vi "Append Control Image to Report.vi"(0 "report in":refnum<class "NI_report.lvclass">, 1 "alignment (default)":T2, 2 "image file type (.jpg)":enum16{".jpg", ".png"}(ring), 5 "image depth":T1=2 items=["B&W", "4 bits", "8 bits", "24 bits"], 7 "ctrl reference":refnum<vi>, 9 "description":string, 11 "error in (no error)":errorcluster, 12 "MS Office parameters":T3) -> (4 "report out":refnum<class "NI_report.lvclass">, 8 "start out (Word)":i32, 10 "end out (Word)":i32, 15 "error out":errorcluster)   [LabVIEW 2017, in "NI_report.lvclass"]
doc: "Creates an image of the front panel object specified in <B>ctrl reference</B> and appends it to a report."
uses:
  <vilib>/Utility/NIReport.llb/NI_report.lvclass
  <vilib>/Utility/NIReport.llb/HTML Report Image Alignment.ctl
  <vilib>/Utility/NIReport.llb/image depth.ctl
  <vilib>/Utility/NIReport.llb/NI_ReportGenerationCore.lvlib
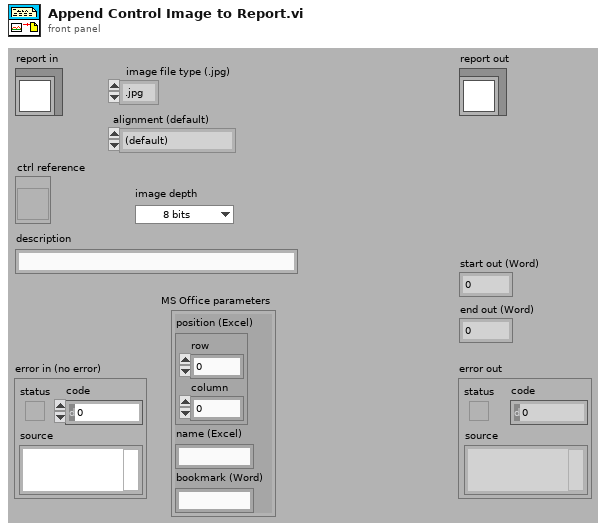
[diagram p1: front panel]
types:
  T1 = typedef "NI_ReportGenerationCore.lvlib/image depth.ctl" = u16
  T2 = typedef "NI_ReportGenerationCore.lvlib/HTML Report Image Alignment.ctl" = enum16{"(default)", "LEFT", "RIGHT", "TOP", "TEXTTOP", "MIDDLE", "ABSMIDDLE", "BASELINE", "BOTTOM", "ABSBOTTOM"}
  T3 = cluster{"position (Excel)":cluster{"row":i32, "column":i32}, "name (Excel)":string, "bookmark (Word)":string}
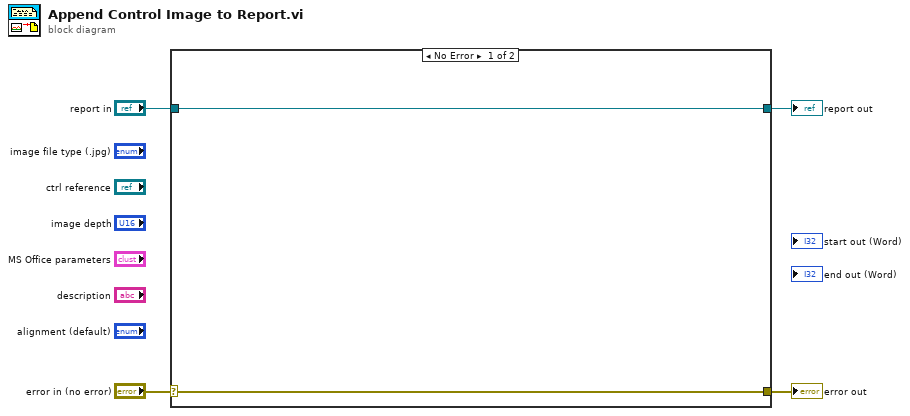
[diagram p0: block diagram]
diagram:
  n1 = case shown="No Error" "error in (no error)" {
    selector: "error in (no error)" -> [w5 w8]
    tunnel: [w5 w8] -> w3
    tunnel: [w6 w7] -> w1
    tunnel: "report in" -> [w6 w7]
    frame No Error {
    }
    frame Error {
    }
  }
  "error out" <- w3
  "report out" <- w1
